vi "Get Sender.vi"(11 "Has Destroyed Msg in":refnum<class "Has Destroyed Msg.lvclass">) -> (2 "Sender":refnum<class "Sender.lvclass">)   [LabVIEW 2020, in "jettl.lvlib" / "Has Destroyed Msg.lvlib" / "Has Destroyed Msg.lvclass"]
uses:
  Has Destroyed Msg.lvclass
  Sender/Sender/Sender.lvclass
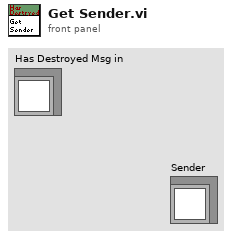
[diagram p1: front panel]
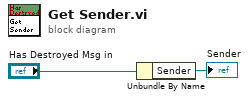
[diagram p0: block diagram]
diagram:
  n1 = Unbundle By Name("Has Destroyed Msg in") -> ("Sender"=→"Sender":refnum<class "Sender.lvclass">)
